vi "Test Trips at 250mA.vi"(3 "error in":errorcluster) -> (10 "error out":errorcluster)   [LabVIEW 2015]
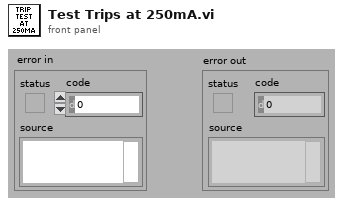
[diagram p1: front panel]
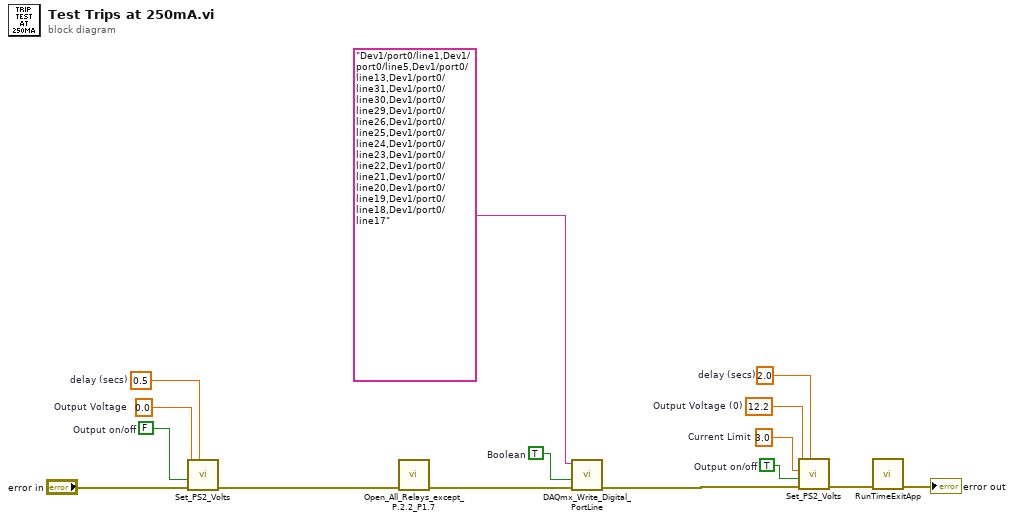
[diagram p0: block diagram]
diagram:
  w3 = 3.0  # Current Limit
  w7 = 0.0  # Output Voltage
  w8 = 0.5  # delay (secs)
  w9 = FALSE  # Output on/off
  w10 = 2.0  # delay (secs)
  w4 = TRUE  # Output on/off
  w13 = 12.2  # Output Voltage (0)
  w15 = TRUE  # Boolean
  n1 = call "Set_PS2_Volts.vi"("delay (secs)"=w8, "error in"="error in", "Output on/off"=w9, "Output Voltage"=w7) -> ("error out"=w5:errorcluster)  [unwired: 5 in, 2 out]
  n2 = call "Open_All_Relays_except_P.2.2_P1.7.vi"("error in"=w5) -> ("error out"=w11:errorcluster)  [unwired: 8 in]
  n3 = call "DAQmx_Write_Digital_PortLine.vi"("Device/Ports/Lines"="Dev1/port0/line1,Dev1/port0/line5,Dev1/port0/line13,Dev1/port0/line31,Dev1/port0/line30,Dev1/port0/line29,Dev1/port0/line26,Dev1/port0/line25,Dev1/port0/line24,Dev1/port0/line23,Dev1/port0/line22,Dev1/port0/line21,Dev1/port0/line20,Dev1/port0/line19,Dev1/port0/line18,Dev1/port0/line17", "Boolean"=w15, "error in"=w11) -> ("error out"=w14:errorcluster)  [unwired: 6 in, 1 out]
  n4 = call "Set_PS2_Volts.vi"("delay (secs)"=w10, "error in"=w14, "Output on/off"=w4, "Current Limit"=w3, "Output Voltage"=w13) -> ("error out"=w2:errorcluster)  [unwired: 4 in, 2 out]
  n5 = call "RunTimeExitApp.vi"("error in (no error)"=w2) -> ("error out"=→"error out":errorcluster)  [unwired: 10 in]
